vi "Pack Launch Nested Views.vi"(10 "View Labels (optional)":string[](array[string]), 11 "Viewables":refnum<class "IViewable.lvclass">[](array[class])) -> (3 "Launch Nested Views Msg":refnum<class "Launch Nested Views Msg.lvclass">)   [LabVIEW 2020, in "Popup ViewManager.lvlib" / "Launch Nested Views Msg.lvclass"]
uses:
  <vilib>/gpm_packages/@cs/popup-viewmanager/Source/Popup ViewManager Messages/Launch Nested Views Msg/Launch Nested Views Msg.lvclass
  <vilib>/gpm_packages/@cs/mva-viewable/Source/IViewable/IViewable/IViewable.lvclass
  <vilib>/gpm_packages/@cs/popup-viewmanager/Source/Popup ViewManager Messages/Launch Nested Views Msg/Launch Nested Views Msg.lvclass/Launch Nested Views Msg.ctl
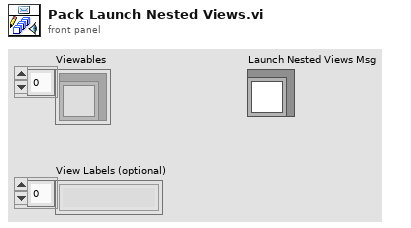
[diagram p1: front panel]
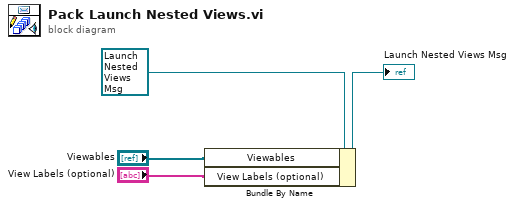
[diagram p0: block diagram]
diagram:
  n1 = Bundle By Name(cluster=refnum<class "Launch Nested Views Msg.lvclass"> refnum ("Popup ViewManager.lvlib:Launch Nested Views Msg.lvclass"), "Viewables"="Viewables", "View Labels (optional)"="View Labels (optional)") -> (→"Launch Nested Views Msg":refnum<class "Launch Nested Views Msg.lvclass">)
